vi "ReadExternalInterfaces.vi"(8 "ErrorIn":errorcluster, 11 "TAFTraceWindow in":refnum<class "TAFTraceWindow.lvclass">) -> (0 "ErrorOut":errorcluster, 2 "ExternalInterfaces":T1[](array[typedef]), 3 "TAFTraceWindow out":refnum<class "TAFTraceWindow.lvclass">)   [LabVIEW 2021]
uses:
  TAFTraceWindow.lvclass
  Library_TAF_Support/ClusterArrayConversion/BundledArray.ctl
  TAFTraceWindow.lvclass/TAFTraceWindow.ctl
  440278e9-1c04-4840-94c9-ed200201a6f0.vi
  C:/Localdata/Projects/TriekselSoft/TriekselsoftApplicationFramework/Source/.Externals/Library_YAF/YAFTAF/YAFTAF.lvclass
  C:/Localdata/Projects/TriekselSoft/TriekselsoftApplicationFramework/Source/.Externals/Library_YAF/YActor/YActor.lvclass
  C:/Localdata/Projects/TriekselSoft/TriekselsoftApplicationFramework/Source/.Externals/Interface_UserInterface_IFrontPanel/IFrontPanel/IFrontPanel.lvclass
  C:/Localdata/Projects/TriekselSoft/TriekselsoftApplicationFramework/Source/IInterface/IInterface.lvclass
  C:/Localdata/Projects/TriekselSoft/TriekselsoftApplicationFramework/Source/.Externals/Interface_Object_ICreateDestroy/ICreateDestroy/ICreateDestroy.lvclass
  C:/Localdata/Projects/TriekselSoft/TriekselsoftApplicationFramework/Source/.Externals/Interface_Object_IPersistentData/IPersistentData/IPersistentData.lvclass
  C:/Localdata/Projects/TriekselSoft/TriekselsoftApplicationFramework/Source/.Externals/Interface_TAF_ITAFObject/ITAFObject/ITAFObject.lvclass
  C:/Localdata/Projects/TriekselSoft/TriekselsoftApplicationFramework/Source/.Externals/Library_TAF_TraceWindow/TAFTraceWindow/TAFTraceWindow.lvclass
  C:/Localdata/Projects/TriekselSoft/TriekselsoftApplicationFramework/Source/.Externals/INewOpenCVMat/INewOpenCVMat.lvclass
  Library_TAF_Support/ClusterArrayConversion/ClusterArrayConversion.lvlib
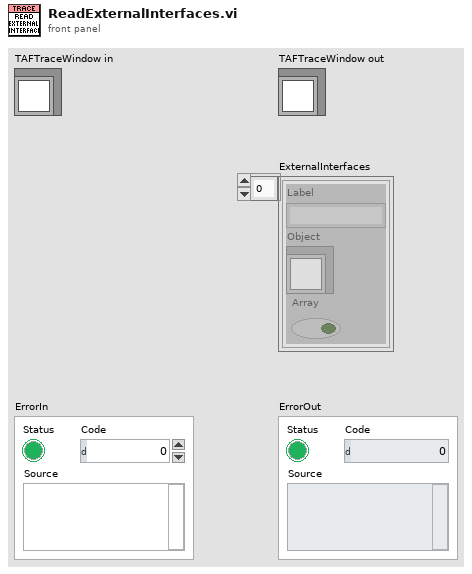
[diagram p1: front panel]
types:
  T1 = typedef "ClusterArrayConversion.lvlib/BundledArray.ctl" = cluster{"Label":string, "Object":refnum<class>, "Array":bool}
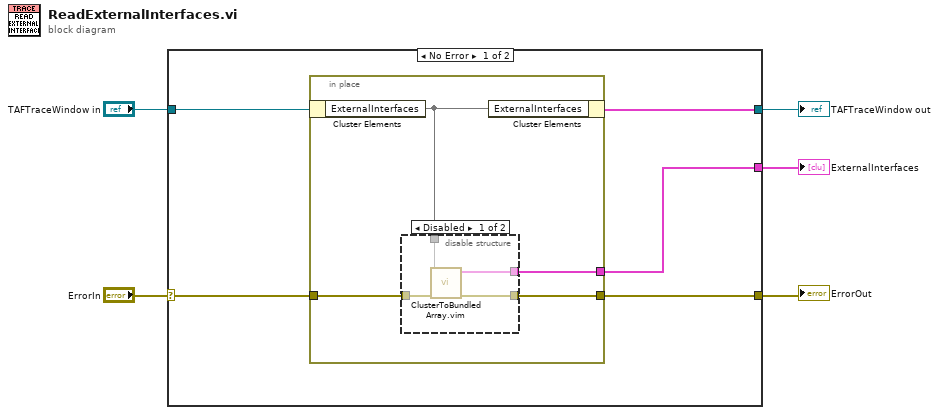
[diagram p0: block diagram]
diagram:
  n1 = case shown="No Error" "ErrorIn" {
    selector: "ErrorIn" -> [w10 w20]
    tunnel: [w9 w20] -> w4
    tunnel: [w7 w19] -> w2
    tunnel: "TAFTraceWindow in" -> [w8 w19]
    tunnel: [w6 _] -> w1
    frame No Error {
      n2 = in-place {
        in-place-border: w10 -> [w14]
        in-place-border: [w13] -> w9
        in-place-border: [w11] -> w6
        n3 = in-place-cluster #1(w8) -> ("ExternalInterfaces"=w12)
        n4 = disable-structure shown="Disabled" {
          disable-tunnel: w14 -> [w18 _]
          disable-tunnel: w12 -> [w16 _]
          disable-tunnel: [w17 _] -> w13
          disable-tunnel: [w15 _] -> w11
          frame Disabled {
            n5 = call "ClusterToBundledArray.vim"("ErrorIn"=w18, "Interfaces"=w16) -> ("ErrorOut"=w17:errorcluster, "BundeledLabels"=w15:T1[])  [unwired: 8 in]
          }
          frame Enabled {
          }
        }
        n6 = in-place-cluster #1("ExternalInterfaces"=w12) -> (w7:cluster{})
      }
    }
    frame Error {
    }
  }
  "ErrorOut" <- w4
  "TAFTraceWindow out" <- w2
  "ExternalInterfaces" <- w1
